vi "Lake Shore Cryotronics 370 Application Configure Reading.vi"() -> ()   [LabVIEW 2024]
doc: "This example vi shows how to configure an input's settings and resistance range and take a resistance reading. The Change Pause time value is used to control the time between configuration and taking the reading. The user is also given the option of not configuring the input and taking a resistance reading only."
uses:
  Lake Shore Cryotronics 370.lvlib
panel:
  in  "VISA resource name":refnum<visa-resource-name>
  in  "Configure (False)":bool
  in  "Temperature Coefficient (0: Negative)":u16(ring) items=["Negative", "Positive"]
  in  "Change Pause Time (3)":dbl=3.0 min=3.0 max=200.0 step=1.0
  in  "Scan Dwell Time (10)":dbl=10.0 min=1.0 max=200.0 step=1.0
  in  "Channel On/Off (T: Channel ON)":bool=TRUE
  in  "Excitation On/Off (T: Excitation ON)":bool=TRUE
  in  "Resistance Range (21: 63.2 MOhm)":u16(ring)=21 items=["2.00 mOhm", "6.32 mOhm", "20.0 mOhm", "63.2 mOhm", "200 mOhm", "632 mOhm", "2.00 Ohm", "6.32 Ohm", "20.0 Ohm", "63.2 Ohm", "200 Ohm", "632 Ohm", "2.00 kOhm", "6.32 kOhm", "20.0 kOhm", "63.2 kOhm", "200 kOhm", "632 kOhm", "2.00 MOhm", "6.32 MOhm", "20.0 MOhm", "63.2 MOhm"]
  in  "Excitation Range (11: 632 mV / 316 nA)":u16(ring)=11 items=["2.00 uV / 1.00 pA", "6.32 uV / 3.16 pA", "20.0 uV / 10.0 pA", "63.2 uV / 31.6 pA", "200 uV / 100 pA", "632 uV / 316 pA", "2.00 mV / 1.00 nA", "6.32 mV / 3.16 nA", "20.0 mV / 10.0 nA", "63.2 mV / 31.6 nA", "200 mV / 100 nA", "632 mV / 316 nA", "1.00 uA", "3.16 uA", "10.0 uA", "31.6 uA", "100 uA", "316 uA", "1.00 mA", "3.16 mA", "10.0 mA", "31.6 mA"]
  in  "Excitation Mode (0: Voltage)":u16(ring) items=["Voltage", "Current"]
  in  "Channel (1)":i32=1 min=0 max=16 step=1
  out "Resistance Reading":dbl min=0.0 max=63200000.0 step=1e-05 format="%^.5e"
  # "(c) 2001 - 2009 National Instruments.  ALL RIGHTS RESERVED."
  # "Channel ON\nChannel OFF"
  # "Excitation ON\nExcitation OFF"
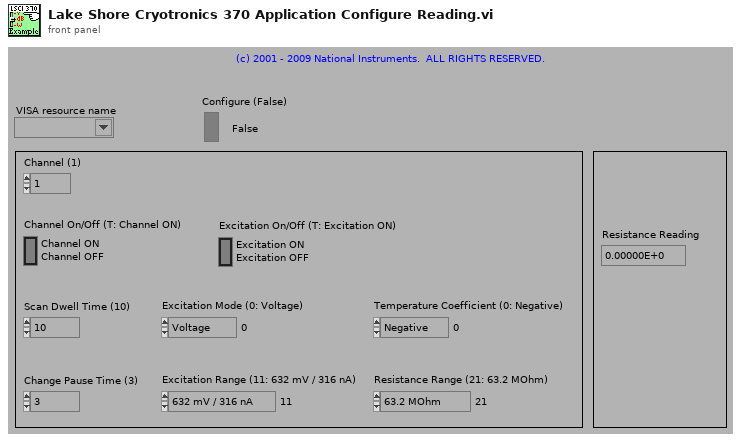
[diagram p1: front panel]
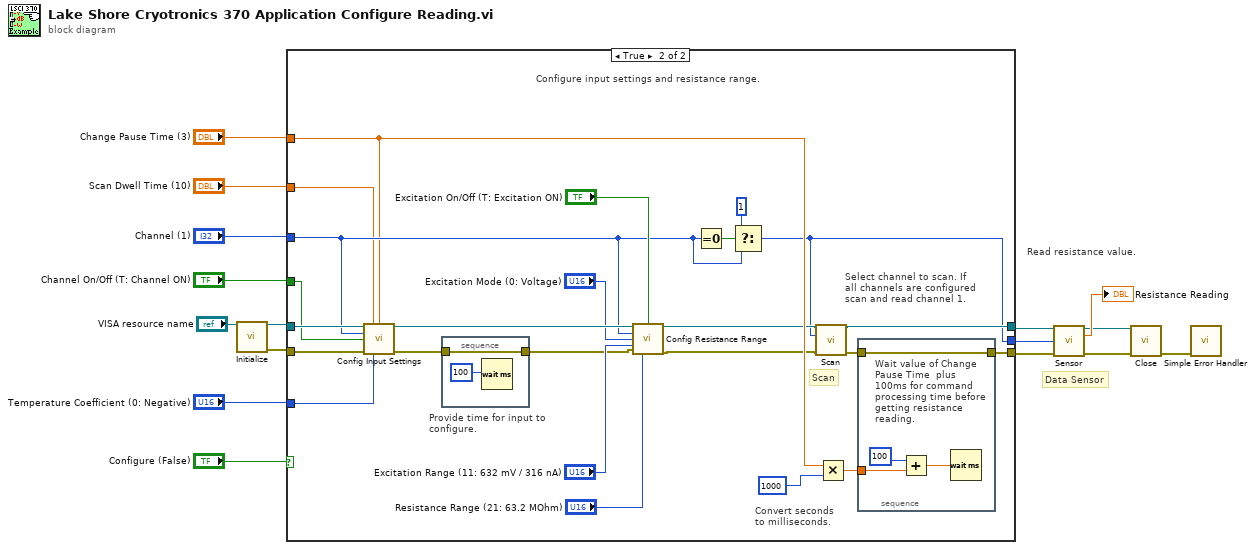
[diagram p0: block diagram]
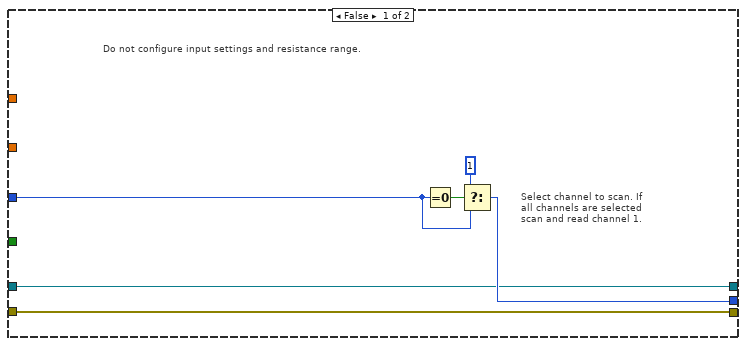
[diagram p2: hidden frame]
diagram:
  # "Data Sensor"
  # "Read resistance value."
  n1 = call "Initialize.vi"("VISA resource name"="VISA resource name") -> ("VISA resource name out"=w16:refnum<visa-resource-name>, "error out"=w15:errorcluster)  [unwired: 13 in]
  n2 = case shown="True" "Configure (False)" {
    tunnel: w15 -> [w17 w46]
    tunnel: w16 -> [w18 w45]
    tunnel: "Channel On/Off (T: Channel ON)" -> [_ w30]
    tunnel: "Scan Dwell Time (10)" -> [_ w28]
    tunnel: "Temperature Coefficient (0: Negative)" -> [_ w43]
    tunnel: [w17 w38] -> w7
    tunnel: [w18 w27] -> w6
    tunnel: "Change Pause Time (3)" -> [_ w29]
    tunnel: "Channel (1)" -> [w19 w33]
    tunnel: [w20 w23] -> w5
    frame False {
      # "Do not configure input settings and resistance range."
      # "Select channel to scan. If\nall channels are selected\nscan and read channel 1."
      n3 = Equal To 0?(x=w19) -> (x = 0?=w22:bool)
      n4 = Select(t=1, s=w22, f=w19) -> (s? t:f=w20:i32)
    }
    frame True {
      # "Scan"
      # "Provide time for input to\nconfigure."
      # "Select channel to scan. If\nall channels are configured\nscan and read channel 1."
      # "Configure input settings and resistance range."
      # "Convert seconds\nto milliseconds."
      n5 = call "Config Input Settings.vi"("VISA resource name"=w45, "Scan Dwell Time (10)"=w28, "Change Pause Time (3)"=w29, "Channel (1)"=w33, "Channel On/Off (T: ON)"=w30, "error in (no error)"=w46, "Temperature Coefficient (0: Negative)"=w43) -> ("VISA resource name out"=w44:refnum<visa-resource-name>, "error out"=w32:errorcluster)  [unwired: 7 in]
      n6 = stacked-sequence {
        tunnel: w32 -> [w47]
        tunnel: [w47] -> w31
        frame #0 {
          n7 = Wait (ms)(milliseconds to wait=100) -> ()  [unwired: 1 out]
        }
      }
      n8 = call "Config Resistance Range.vi"("VISA resource name"=w44, "Excitation  (T: On)"="Excitation On/Off (T: Excitation ON)", "Channel (1)"=w33, "Excitation Mode (0: Voltage)"="Excitation Mode (0: Voltage)", "Excitation Range (11: 632 mV / 316 nA)"="Excitation Range (11: 632 mV / 316 nA)", "error in (no error)"=w31, "Resistance Range (21: 63.2 MOhm)"="Resistance Range (21: 63.2 MOhm)") -> ("VISA resource name out"=w24:refnum<visa-resource-name>, "error out"=w25:errorcluster)  [unwired: 7 in]
      n9 = Equal To 0?(x=w33) -> (x = 0?=w35:bool)
      n10 = Select(t=1, s=w35, f=w33) -> (s? t:f=w23:i32)
      n11 = call "Scan.vi"("VISA resource name"=w24, "Scan Channel (1)"=w23, "error in (no error)"=w25) -> ("VISA resource name out"=w27:refnum<visa-resource-name>, "error out"=w26:errorcluster)  [unwired: 11 in]
      n12 = Multiply(x=w29, y=1000) -> (x*y=w36:dbl)
      n13 = stacked-sequence {
        tunnel: w26 -> [w52]
        tunnel: [w52] -> w38
        tunnel: w36 -> [w50]
        frame #0 {
          # "Wait value of Change\nPause Time  plus \n100ms for command\nprocessing time before\ngetting resistance \nreading."
          n14 = Add(x=100, y=w50) -> (x+y=w49:dbl)
          n15 = Wait (ms)(milliseconds to wait=w49) -> ()  [unwired: 1 out]
        }
      }
    }
  }
  n16 = call "Sensor.vi"("VISA resource name"=w6, "Channel (1)"=w5, "error in (no error)"=w7) -> ("VISA resource name out"=w2:refnum<visa-resource-name>, "Resistance Reading"=→"Resistance Reading":dbl, "error out"=w3:errorcluster)  [unwired: 8 in, 2 out]
  n17 = call "Close.vi"("VISA resource name"=w2, "error in (no error)"=w3) -> ("error out"=w1:errorcluster)  [unwired: 13 in]
  n18 = call <vilib>:"Simple Error Handler.vi"("error in (no error)"=w1) -> ()  [unwired: 4 in, 5 out]
